vi "RunningAverage-AddSection.vi"(8 "Error in":errorcluster, 10 "CD Settings in":T1 {"CD Task Dependency Ref" format="%.0x"; "CD Task Dependency" format="%.0x"}, 11 "Custom Device ref":T2 format="%.0x") -> (0 "Error out":errorcluster, 3 "Custom Device ref out":T2 format="%.0x")   [LabVIEW 2017, in "Waveform-Processing-Custom-Device Shared.lvlib" / "Running Average.lvlib"]
uses:
  Running Average.lvlib
  <vilib>/NI Veristand/Custom Device API/Custom Device Item Ref.ctl
  Custom Device Settings.ctl
  <vilib>/NI Veristand/Custom Device API/Custom Device Channel.ctl
  <vilib>/NI Veristand/Custom Device API/Custom Device Channel Type.ctl
  Constants.vi
  <vilib>/NI Veristand/Custom Device API/Set Item Property (Dependent Node Pointer).vi
  Waveform-Processing-Custom-Device Shared.lvlib
  <vilib>/NI Veristand/Custom Device API/Custom Device API.lvlib
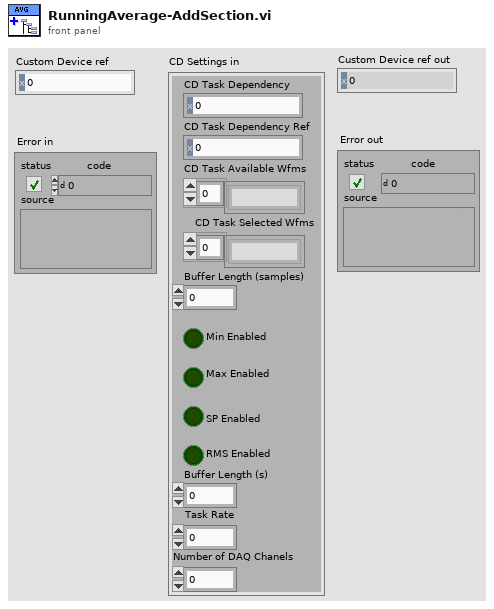
[diagram p1: front panel]
types:
  T1 = typedef "Waveform-Processing-Custom-Device Shared.lvlib/Custom Device Settings.ctl" = cluster{"CD Task Dependency":T2, "CD Task Dependency Ref":T2, "CD Task Available Wfms":string[], "CD Task Selected Wfms":string[], "Buffer Length (samples)":u32, "Min Enabled":bool, "Max Enabled ":bool, "SP Enabled":bool, "RMS Enabled":bool, "Buffer Length (s)":dbl, "Task Rate":dbl, "Number of DAQ Chanels":u32}
  T2 = typedef "Custom Device API.lvlib/Custom Device Item Ref.ctl" = u64
  T3 = typedef "Custom Device API.lvlib/Custom Device Channel Type.ctl" = enum16{"Input", "Output"}
  T4 = typedef "Custom Device API.lvlib/Custom Device Channel.ctl" = cluster{"Type":T3, "Units":string, "Default Value":dbl, "Faultable":bool, "Scalable":bool}
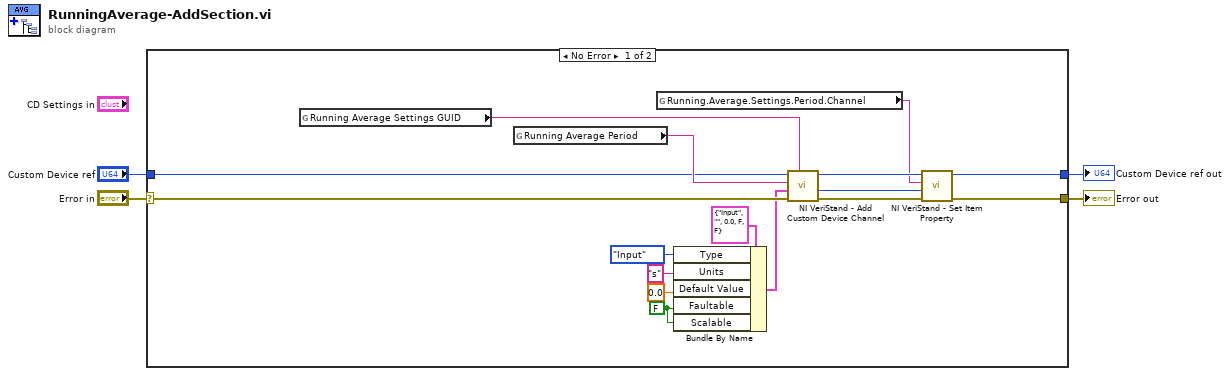
[diagram p0: block diagram]
diagram:
  n1 = case shown="No Error" "Error in" {
    selector: "Error in" -> [w20 w22]
    tunnel: "Custom Device ref" -> [w6 w21]
    tunnel: [w14 w22] -> w2
    tunnel: [w5 w21] -> w1
    frame No Error {
      w8 = FALSE ("Faultable")
      n2 = global read "Constants.vi" "Running Average Settings GUID"() -> (w7:string)
      n3 = global read "Constants.vi" "Running Average Period"() -> (w19:string)
      n4 = global read "Constants.vi" "Running.Average.Settings.Period.Channel"() -> (w15:string)
      n5 = Bundle By Name(cluster=T4 {"Type"=enum."Input", "Units"="", "Default Value"=0.0, "Faultable"=FALSE, "Scalable"=FALSE} ("Channel"), "Type"=Custom_Device_Channel_Type."Input", "Units"="s", "Default Value"=0.0, "Faultable"=w8, "Scalable"=w8) -> (w12:T4)
      n6 = call <vilib>:"NI VeriStand - Add Custom Device Channel.vi"("GUID (Default Channel)"=w7, "error in (no error)"=w20, "Channel"=w12, "Channel Name"=w19, "Parent Ref in"=w6) -> ("error out"=w16:errorcluster, "Channel Ref"=w17:T2, "Parent Ref out"=w18:T2)  [unwired: 3 in, 1 out]
      n7 = call-poly <vilib>:"NI VeriStand - Set Item Property.vi"("error in (no error)"=w16, "Dependent Node Ref"=w17, "Property Name"=w15, "Item Ref in"=w18) -> ("error out"=w14:errorcluster, "Item Ref out"=w5:T2)  [unwired: 5 in, 1 out]
    }
    frame Error {
    }
  }
  "Error out" <- w2
  "Custom Device ref out" <- w1
